vi "CLUSTER AGE.vi"() -> ()   [LabVIEW 2018]
panel:
  out "output cluster":T1
  in  "Cluster":T2
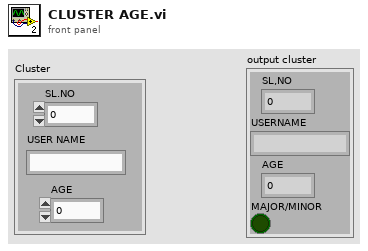
[diagram p1: front panel]
types:
  T1 = cluster{"SL,NO":i32, "USERNAME":string, "AGE":i32, "MAJOR/MINOR":bool}
  T2 = cluster{"SL.NO":i32, "USER NAME":string, "AGE":i32}
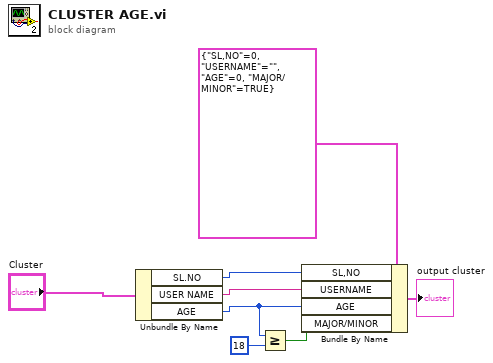
[diagram p0: block diagram]
diagram:
  n1 = Unbundle By Name("Cluster") -> ("SL.NO"=w5:i32, "USER NAME"=w7:string, "AGE"=w3:i32)
  n2 = Greater Or Equal?(x=w3, y=18) -> (x >= y?=w4:bool)
  n3 = Bundle By Name(cluster=T1 {"SL,NO"=0, "USERNAME"="", "AGE"=0, "MAJOR/MINOR"=TRUE}, "SL,NO"=w5, "USERNAME"=w7, "AGE"=w3, "MAJOR/MINOR"=w4) -> (→"output cluster":T1)
